vi "run_chatcompletion_core.vi"(0 "chatcompletion_llm_interface in":refnum<class "llm_gemini_chatmodels.lvclass">, 5 "Messages":refnum<class "abstract_message_base.lvclass">[](array[class]), 11 "error in (no error)":errorcluster) -> (4 "chatcompletion_llm_interface out":refnum<class "llm_gemini_chatmodels.lvclass">, 6 "Response":refnum<class "abstract_message_base.lvclass">, 15 "error out":errorcluster)   [LabVIEW 2020, in "llm_gemini_chatmodels.lvclass"]
uses:
  llm_gemini_chatmodels.lvclass
  abstract_message_base/abstract_message_base.lvclass
  message_text/message_text.lvclass
  C:/Users/venkatesh.chandragir/Downloads/labview-llm-libraries-users-nigharikkha-vlm_support/src/models/abstract_message_base/abstract_message_base.lvclass
  message_text/message.ctl
  <vilib>/httpClient/POSTBuffer.vi
  <vilib>/httpClient/LabVIEWHTTPClient.lvlib
panel:
  out "body":string
  out "headers":string
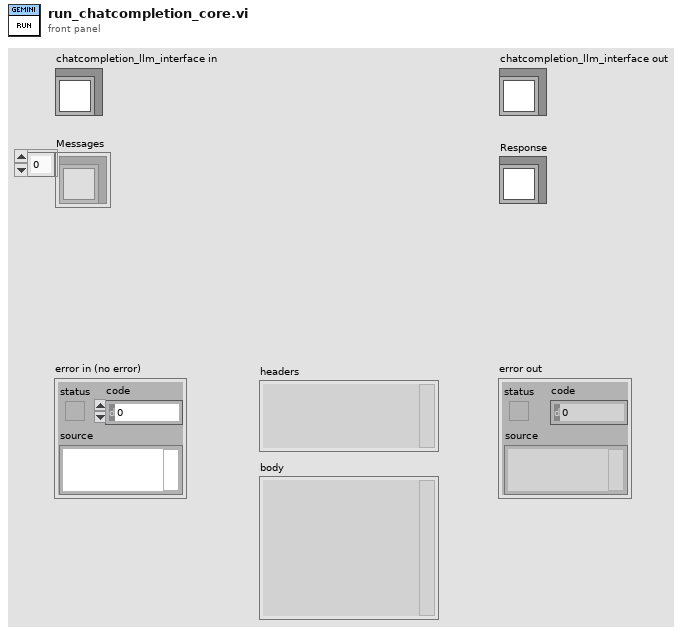
[diagram p1: front panel]
types:
  T1 = typedef "message_text.lvclass/message.ctl" = cluster{"role":string, "content":string[]}
  T2 = typedef "LabVIEWHTTPClient.lvlib/ClientHandle.ctl" = refnum<k1>
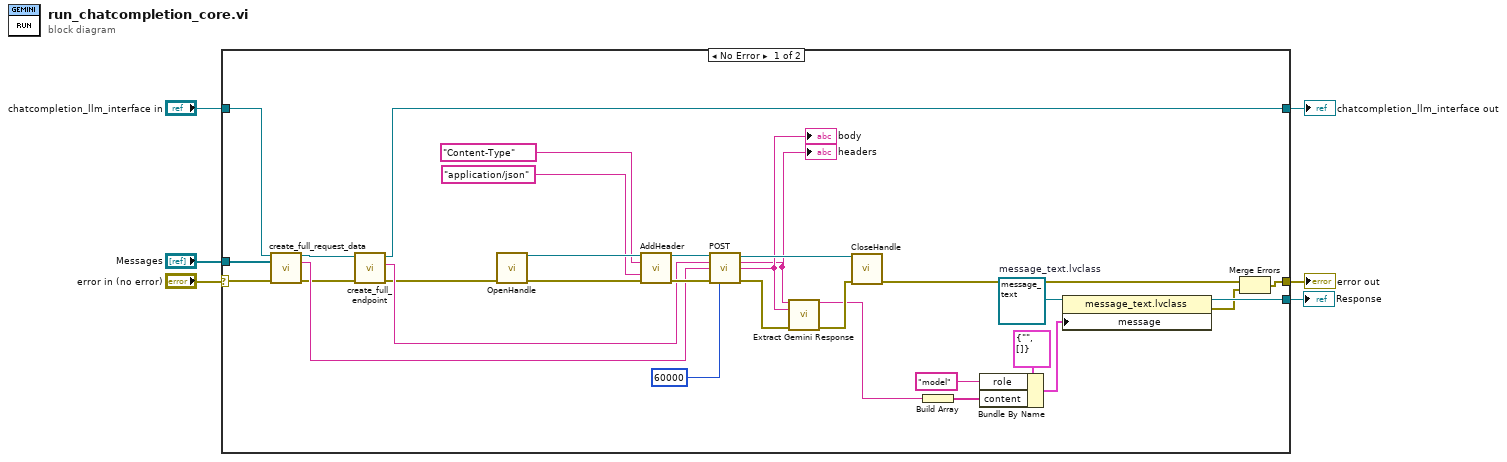
[diagram p0: block diagram]
diagram:
  n1 = case shown="No Error" "error in (no error)" {
    selector: "error in (no error)" -> [w22 w39]
    tunnel: [w25 w39] -> w5
    tunnel: "chatcompletion_llm_interface in" -> [w24 w38]
    tunnel: [w16 w38] -> w3
    tunnel: "Messages" -> [w23 _]
    tunnel: [w8 _] -> w1
    frame No Error {
      w14 = refnum<class "message_text.lvclass"> refnum  # message_text.lvclass
      n2 = call-dynamic "create_full_request_data.vi"("llm_openai_chatmodels in"=w24, "Messages"=w23, "error in (no error)"=w22) -> ("llm_openai_chatmodels out"=w20:refnum<class "llm_gemini_chatmodels.lvclass">, "Request Data"=w21:string, "error out"=w19:errorcluster)  [unwired: 10 in]
      n3 = call-dynamic "create_full_endpoint.vi"("error in (no error)"=w19, "llm_openai_chatmodels in"=w20) -> ("error out"=w17:errorcluster, "endpoint"=w18:string, "llm_openai_chatmodels out"=w16:refnum<class "llm_gemini_chatmodels.lvclass">)  [unwired: 7 in]
      n4 = call <vilib>:"OpenHandle.vi"("error in (no error)"=w17) -> ("client handle out"=w37:T2, "error out"=w36:errorcluster)  [unwired: 13 in]
      n5 = call <vilib>:"AddHeader.vi"("client handle"=w37, "header"="Content-Type", "value"="application/json", "error in (no error)"=w36) -> ("client handle out"=w33:T2, "error out"=w32:errorcluster)  [unwired: 10 in]
      n6 = call-poly <vilib>:"POST.vi"("client handle"=w33, "url"=w18, "buffer"=w21, "error in (no error)"=w32, "timeout (10000)"=60000) -> ("client handle out"=w30:T2, "headers"=w26:string, "body"=w27:string, "error out"=w29:errorcluster)  [unwired: 7 in]
      "headers" <- w26
      "body" <- w27
      n7 = call "Extract Gemini Response.vi"("headers"=w26, "body"=w27, "error in"=w29) -> ("value"=w10:string, "error out"=w28:errorcluster)  [unwired: 11 in]
      n8 = call <vilib>:"CloseHandle.vi"("client handle"=w30, "error in (no error)"=w28) -> ("error out"=w31:errorcluster)  [unwired: 13 in]
      n9 = Build Array(w10) -> (w11:string[])
      n10 = Bundle By Name(cluster=T1 {"role"="", "content"=[]} ("message"), "role"="model", "content"=w11) -> (w9:T1)
      n11 = property class="message_text.lvclass"(reference=w14, "message"=w9) -> (reference out=w8:refnum<class "message_text.lvclass">, error out=w7:errorcluster)  [unwired: 1 in]
      n12 = Merge Errors(w31, w7) -> (w25:errorcluster)
    }
    frame Error {
    }
  }
  "error out" <- w5
  "chatcompletion_llm_interface out" <- w3
  "Response" <- w1
